vi "CSM MDI.vi"(7 "Name (\"\" to Use UUID)":string="Event CSM") -> ()   [LabVIEW 2020, in "MDI ViewManager.lvlib"]
uses:
  MDI ViewManager.lvlib
  Typedef/View.ctl
  <vilib>/Utility/miscctls.llb/LVPointTypeDef.ctl
  <vilib>/Utility/miscctls.llb/LVPoint32TypeDef.ctl
  Typedef/Layout.ctl
  <vilib>/Utility/miscctls.llb/LVBoundsTypeDef.ctl
  <vilib>/Utility/miscctls.llb/LVPositionTypeDef.ctl
  Typedef/Update View.ctl
  e08e3f9e-33cf-4499-bbf1-3a0f395d34a1.vi
  81b46446-0aca-48f9-86dc-ebdbbb8ef4b6.vi
  7ba8cf38-d999-4af7-9cb2-e6092c4454ab.vi
  5110686f-90b8-48a6-8112-abce107b1655.vi
  <userlib>/_NEVSTOP/Communicable State Machine(CSM)/AdvanceAPI/CSM - Revert Arguments-Safe String.vi
  <userlib>/_NEVSTOP/Communicable State Machine(CSM)/_Shared/Trim Single-line Text.vi
  <userlib>/_NEVSTOP/Communicable State Machine(CSM)/AdvanceAPI/CSM - Make String Arguments Safe.vi
  <userlib>/_NEVSTOP/Communicable State Machine(CSM)/AdvanceAPI/CSM - Break Down Multiple States String.vi
  <userlib>/_NEVSTOP/Communicable State Machine(CSM)/AdvanceAPI/CSM - Compact Multiple States.vi
  e08e3f9e-33cf-4499-bbf1-3a0f395d34a1.vi/b09b9099-6be0-413b-8afc-4908471460c3.vi
  <userlib>/_NEVSTOP/Communicable State Machine(CSM)/addons/INI-Static-Variable-Support/_Support/FlagInstance-CSMINIVariable.vi
  81b46446-0aca-48f9-86dc-ebdbbb8ef4b6.vi/99de0c97-112a-4c86-9094-c187659127e1.vi
  <userlib>/_NEVSTOP/Communicable State Machine(CSM)/AdvanceAPI/CSM - Keywords.vi
  <userlib>/_NEVSTOP/Communicable State Machine(CSM)/_Support/ChangeFlag/ChangeFlag-Read.vi
  <vilib>/Utility/cursorutil.llb/Set Cursor (Icon Pict).vi
  <userlib>/_NEVSTOP/Communicable State Machine(CSM)/_Support/ChangeFlag/ChangeFlagDB.vi
  <vilib>/Utility/Data Type/Get Type Information.vi
  <userlib>/_NEVSTOP/Communicable State Machine(CSM)/addons/API-String-Arugments-Support/_Support/Data To SingleElementsArray_csm.vi
  <userlib>/_NEVSTOP/Communicable State Machine(CSM)/addons/INI-Static-Variable-Support/_Support/Parse Used Session and Name.vi
  <userlib>/_NEVSTOP/Communicable State Machine(CSM)/addons/API-String-Arugments-Support/_Support/Data To API String Arguments.vi
  <userlib>/_NEVSTOP/Communicable State Machine(CSM)/addons/INI-Static-Variable-Support/_Support/INI-FGV(lvlibp).vi
  <userlib>/_NEVSTOP/Communicable State Machine(CSM)/addons/INI-Static-Variable-Support/_Support/Populate String with INI Variable.vi
  <userlib>/_NEVSTOP/Communicable State Machine(CSM)/addons/API-String-Arugments-Support/_Support/Convert API String Arguments to Data(variant).vi
  <userlib>/_NEVSTOP/Communicable State Machine(CSM)/addons/API-String-Arugments-Support/_Support/SingleElementsArray To Data_csm.vi
  <userlib>/_NEVSTOP/Communicable State Machine(CSM)/Communicable State Machine.lvlib
  <userlib>/_NEVSTOP/Communicable State Machine(CSM)/addons/INI-Static-Variable-Support/INI-Static-Variable-Support.lvlib
panel:
  in  "Tab Control 40":T1 caption="View0"
  in  "Tab Control 39":T1 caption="View1"
  in  "Tab Control 38":T1 caption="View2"
  in  "Tab Control 37":T1 caption="View3"
  in  "Tab Control 36":T1 caption="View4"
  in  "Tab Control 35":T1 caption="View5"
  in  "Tab Control 34":T1 caption="View6"
  in  "Tab Control 33":T1 caption="View7"
  in  "Tab Control 32":T1 caption="View8"
  in  "Tab Control 31":T1 caption="View9"
  in  "Tab Control 30":T1 caption="View10"
  in  "Tab Control 29":T1 caption="View11"
  in  "Tab Control 28":T1 caption="View12"
  in  "Tab Control 27":T1 caption="View13"
  in  "Tab Control 26":T1 caption="View14"
  in  "Tab Control 25":T1 caption="View15"
  in  "Tab Control 24":T1 caption="View16"
  in  "Tab Control 23":T1 caption="View17"
  in  "Tab Control 22":T1 caption="View18"
  in  "Tab Control 21":T1 caption="View19"
  in  "Tab Control 20":T1 caption="View20"
  in  "Tab Control 19":T1 caption="View21"
  in  "Tab Control 18":T1 caption="View22"
  in  "Tab Control 17":T1 caption="View23"
  in  "Tab Control 16":T1 caption="View24"
  in  "Tab Control 15":T1 caption="View25"
  in  "Tab Control 14":T1 caption="View26"
  in  "Tab Control 13":T1 caption="View27"
  in  "Tab Control 12":T1 caption="View28"
  in  "Tab Control 11":T1 caption="View29"
  in  "Tab Control 10":T1 caption="View30"
  in  "Tab Control 9":T1 caption="View31"
  in  "Tab Control 8":T1 caption="View32"
  in  "Tab Control 7":T1 caption="View33"
  in  "Tab Control 6":T1 caption="View34"
  in  "Tab Control 5":T1 caption="View35"
  in  "Tab Control 4":T1 caption="View36"
  in  "Tab Control 3":T1 caption="View37"
  in  "Tab Control 2":T1 caption="View38"
  in  "Tab Control":T1 caption="View39"
  out "State History":string
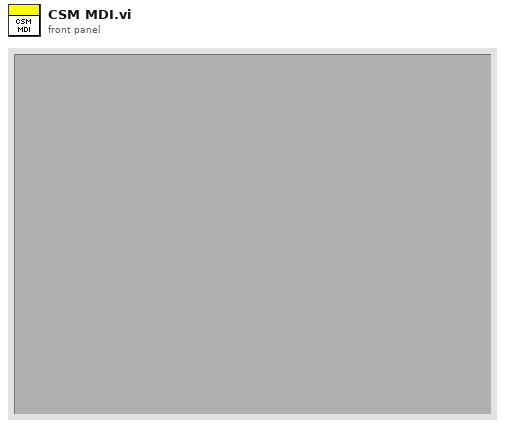
[diagram p1: front panel]
types:
  T1 = typedef "MDI ViewManager.lvlib/View.ctl" = enum32{"Page 1", "Page 2"}
  T2 = typedef "LVPointTypeDef.ctl" = cluster{"Horizontal":i16, "Vertical":i16}
  T3 = typedef "LVPoint32TypeDef.ctl" = cluster{"Horizontal":i32, "Vertical":i32}
  T4 = typedef "MDI ViewManager.lvlib/Layout.ctl" = cluster{"Origin":T2, "Layout":cluster{"Pane Dimension":T5, "Position":T6, "Label":string, "Visible":bool, "InsertedViewName":string}[]}
  T5 = typedef "LVBoundsTypeDef.ctl" = cluster{"Width":u32, "Height":u32}
  T6 = typedef "LVPositionTypeDef.ctl" = cluster{"Left":i32, "Top":i32}
  T7 = typedef "MDI ViewManager.lvlib/Update View.ctl" = cluster{"Name":string, "VIPath":path, "Height(Default)":u32, "Widht(Default)":u32, "VIRef":refnum<vi>}
  T8 = cluster{"Ref":cluster{"TabCtls":refnum<vi>[], "CurrMoveCtl":refnum<vi>, "Pane":refnum<vi>, "SubPanel":refnum<vi>, "Owning VI":refnum<vi>}, "Val":cluster{"TabCtlMove?":bool, "MouseOffset":T3, "LayoutMap":map{string, T4}, "ViewMap":map{string, T7}}}
  T9 = cluster{"Current VI Reference":refnum<vi>, "Close Panel on Exit?":bool}
  T10 = cluster{"Core":cluster{"Current VI Reference":refnum<vi>, "Close Panel on Exit?":bool}, "1":cluster{"Ref":cluster{"TabCtls":refnum<vi>[], "CurrMoveCtl":refnum<vi>, "Pane":refnum<vi>, "SubPanel":refnum<vi>, "Owning VI":refnum<vi>}, "Val":cluster{"TabCtlMove?":bool, "MouseOffset":T3, "LayoutMap":map{string, T4}, "ViewMap":map{string, T7}}}}
  T11 = enum32{"Invalid", "Standard", "Closed", "Hidden", "Minimized", "Maximized"}
  T12 = enum32{"invalid app kind", "Development System", "Run Time System", "Student Edition", "Embedded LabVIEW", "Evaluation", "Custom"}
  T13 = cluster{"TabCtl":refnum<vi>[], "Pane":refnum<vi>, "Variant":variant, "map in":map{string, T4}}
  T14 = cluster{"Pane":refnum<vi>, "TabCtls":refnum<vi>[], "map in":map{string, T4}, "Views":map{string, T7}}
  T15 = typedef "Communicable State Machine.lvlib/_CSM_Response Source Message.ctl" = cluster{"‘State":string, "’Arguments":string, "’Error":errorcluster}
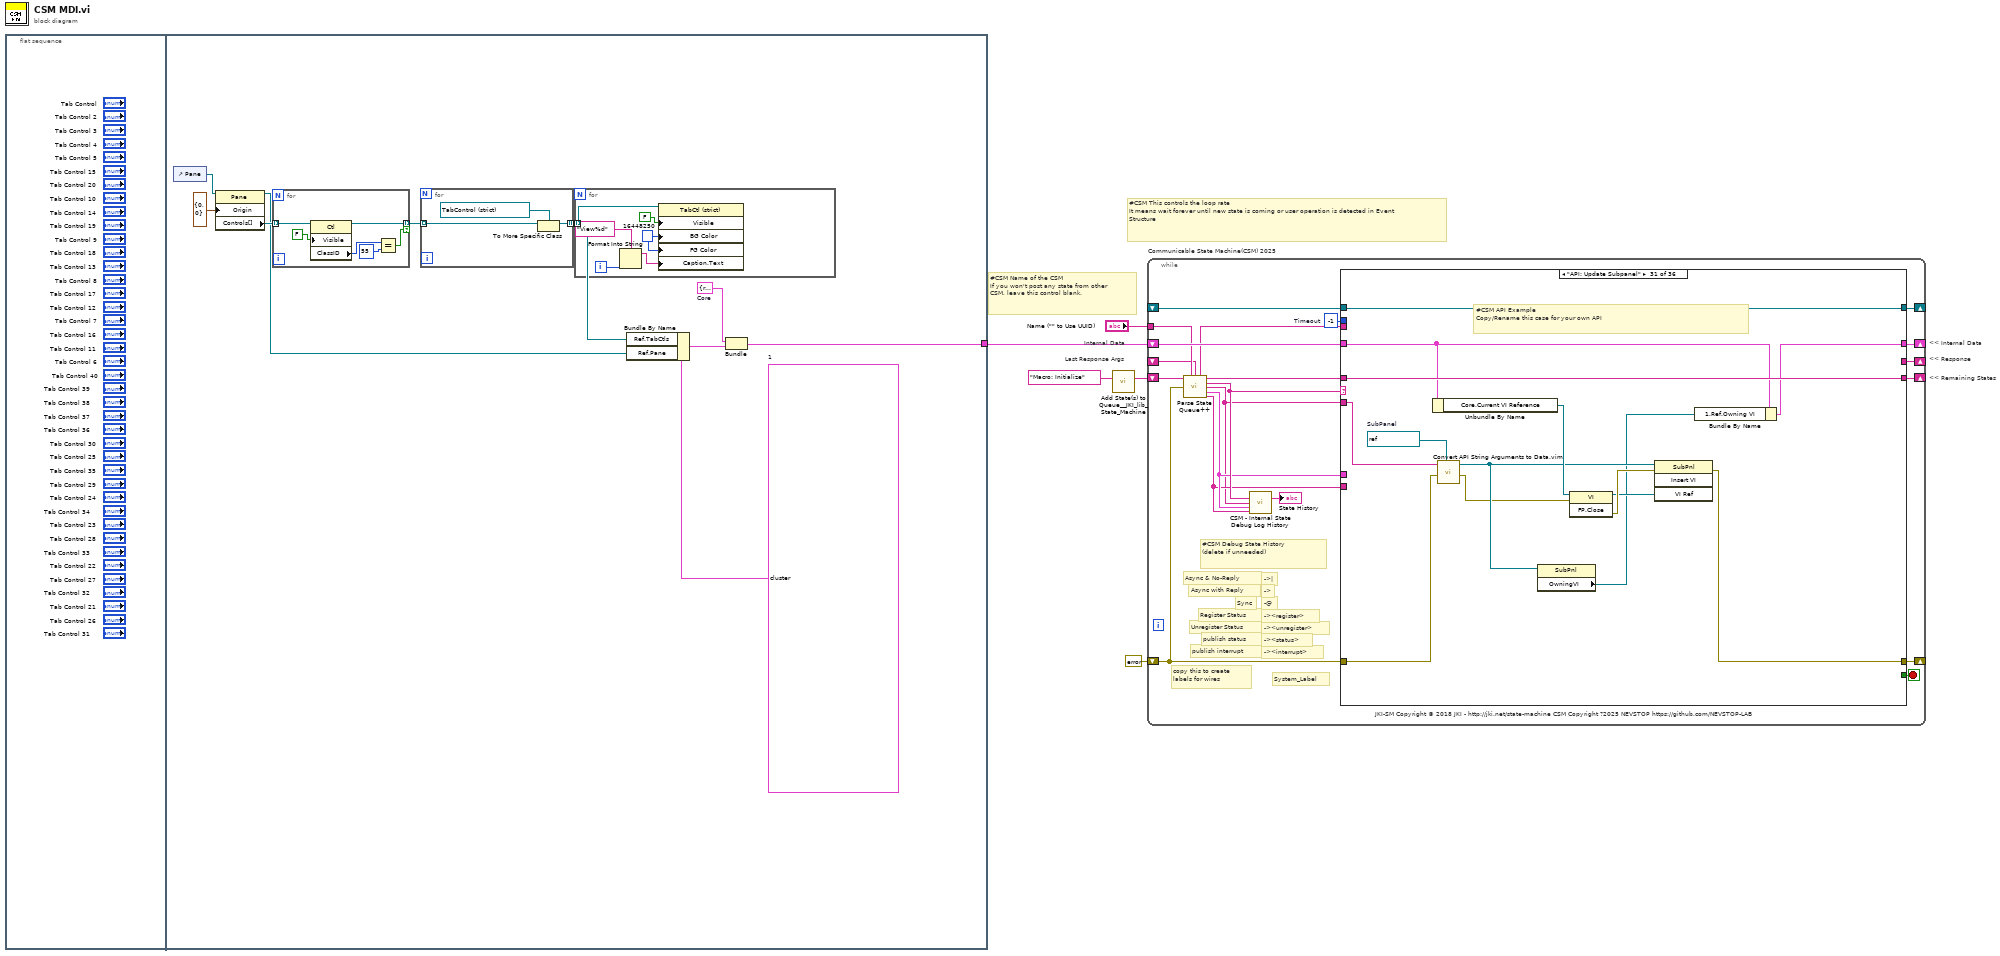
[diagram p0: block diagram]
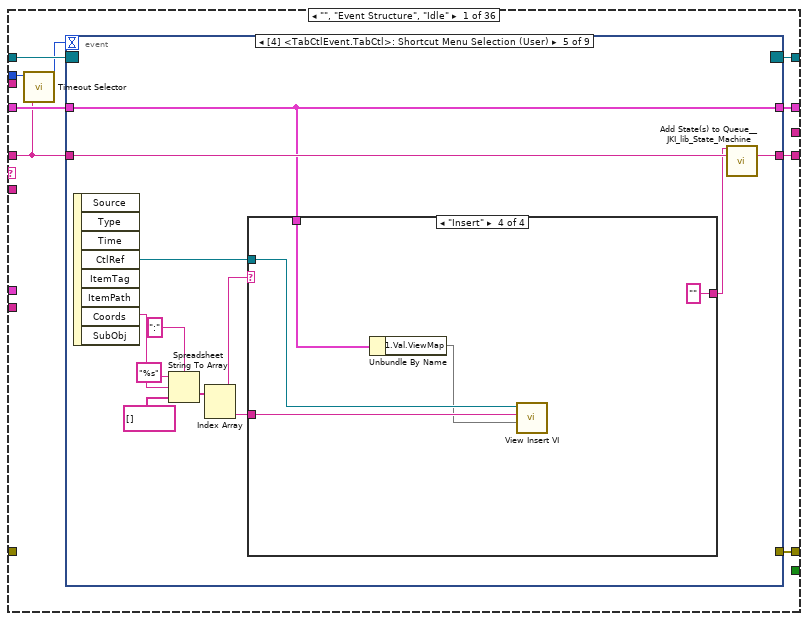
[diagram p2: hidden frame]
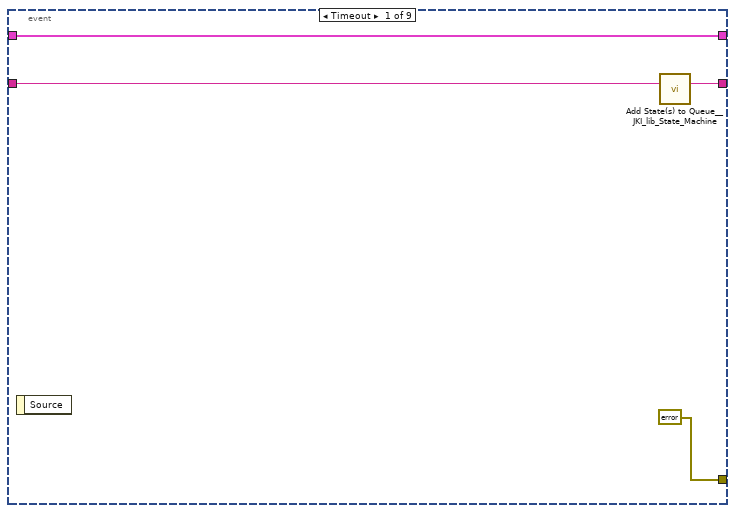
[diagram p3: hidden frame]
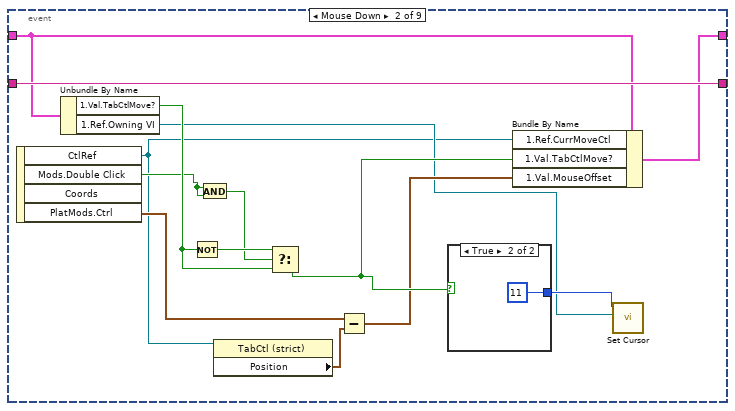
[diagram p4: hidden frame]
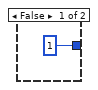
[diagram p5: hidden frame]
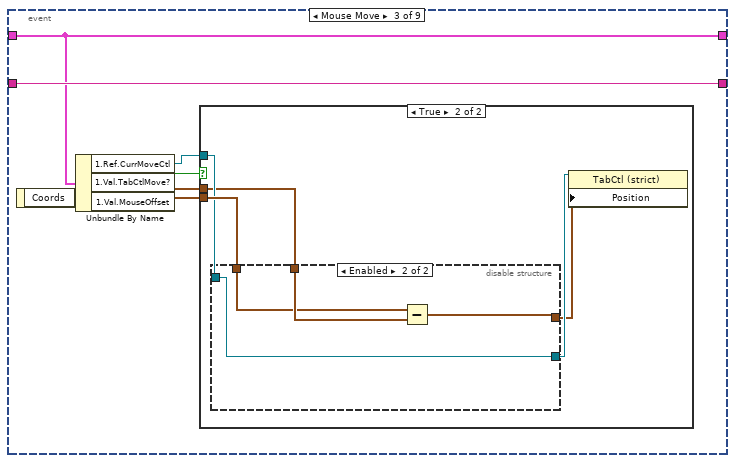
[diagram p6: hidden frame]
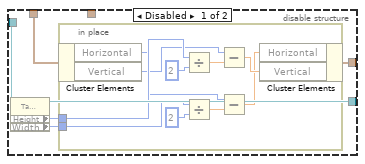
[diagram p8: hidden frame]
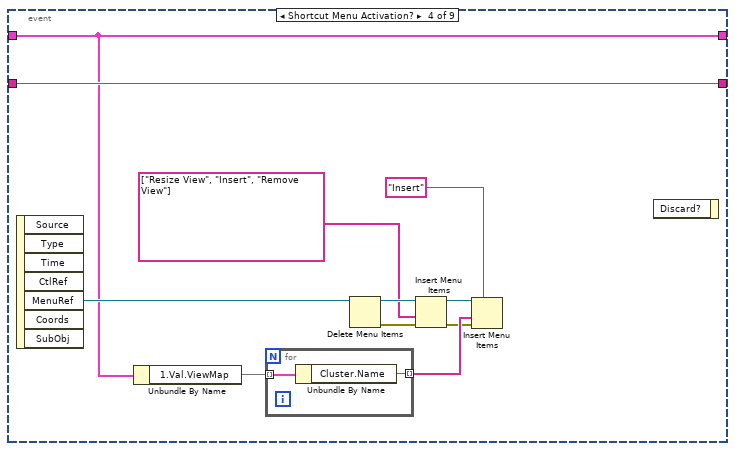
[diagram p9: hidden frame]
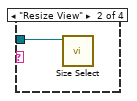
[diagram p11: hidden frame]
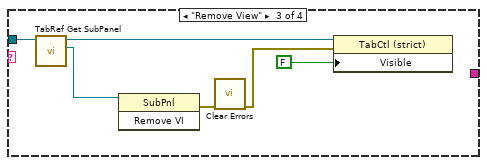
[diagram p12: hidden frame]
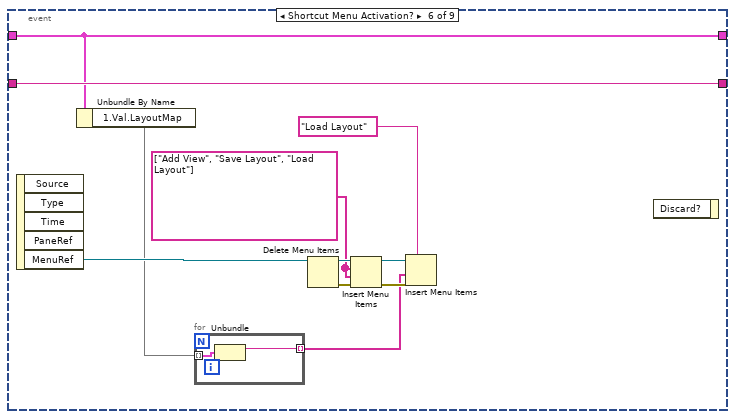
[diagram p13: hidden frame]
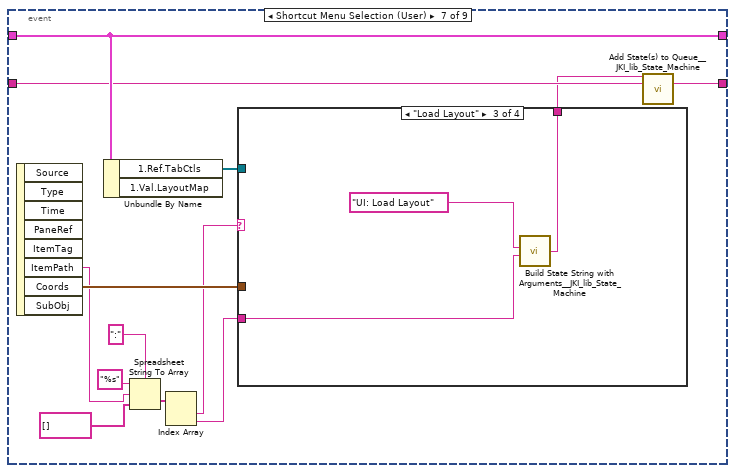
[diagram p14: hidden frame]
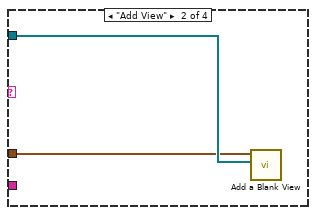
[diagram p16: hidden frame]
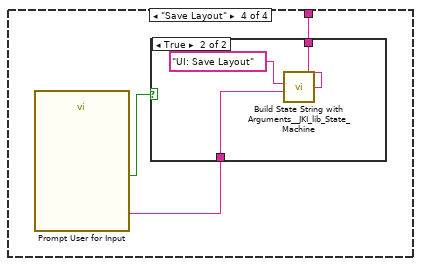
[diagram p17: hidden frame]
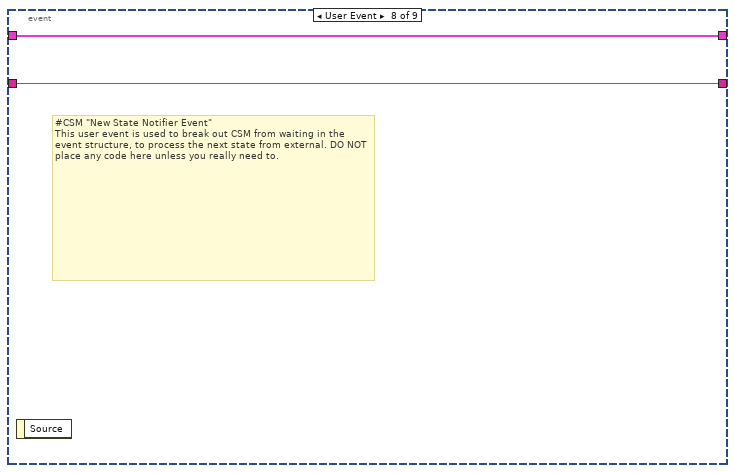
[diagram p19: hidden frame]
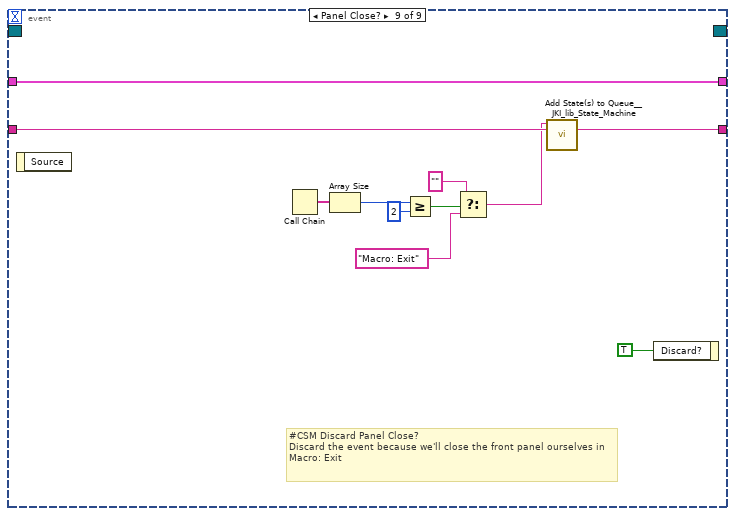
[diagram p20: hidden frame]
diagram:
  # "Last Response Args"
  # "Internal Data"
  # "<< Internal Data"
  # "<< Response"
  # "<< Remaining States"
  # "#CSM Name of the CSM\nIf you won't post any state from other CSM, leave this control blank."
  # "#CSM This controls the loop rate\nIt means wait forever until new state is coming or user operation is detected in Event Structure"
  n1 = flat-sequence {
    tunnel: [w15] -> w1
    frame #0 {
    }
    frame #1 {
      w13 = T8 {"Ref"={"TabCtls"=[], "CurrMoveCtl"=refnum, "Pane"=refnum, "SubPanel"=refnum, "Owning VI"=refnum}, "Val"={"TabCtlMove?"=FALSE, "MouseOffset"={"Horizontal"=0, "Vertical"=0}, "LayoutMap"={}, "ViewMap"={}}}  # 1
      w12 = T9 {"Current VI Reference"=refnum, "Close Panel on Exit?"=FALSE}  # Core
      n2 = control-ref of="Pane"() -> (w9:refnum<vi>)
      n3 = property class="Pane"(reference=w9, "Origin"=T2 {"Horizontal"=0, "Vertical"=0}) -> (reference out=w6:refnum<vi>, "Controls[]"=w10:refnum<vi>[])  [unwired: 1 in, 1 out]
      n4 = for {
        tunnel: w10 -> [w24] mode=indexing
        tunnel: [w19] -> w8 mode=indexing if=w20
        n5 = property class="Ctl"(reference=w24, "Visible"=FALSE) -> (reference out=w19:refnum<vi>, "ClassID"=w22:u32)  [unwired: 1 in, 1 out]
        n6 = Equal?(x=w22, y=u32 55) -> (x = y?=w20:bool)
      }
      n7 = for {
        tunnel: w8 -> [w18] mode=indexing
        tunnel: [w17] -> w7 mode=indexing
        n8 = To More Specific Class(target class=refnum<vi> refnum ("Tab Control"), reference=w18) -> (specific class reference=w17:refnum<vi>)  [unwired: 1 in, 1 out]
      }
      n9 = for {
        tunnel: w7 -> [w29] mode=indexing
        i -> [w27]
        w28 = u32 16448250 ("Colors:BG Color")
        n10 = Format Into String(format string="View%d", w27) -> (resulting string=w26:string)  [unwired: 2 in, 1 out]
        n11 = property class="TabCtl (strict)"(reference=w29, "Visible"=FALSE, "BG Color"=w28, "FG Color"=w28, "Caption.Text"=w26) -> ()  [unwired: 1 in, 2 out]
      }
      n12 = Bundle By Name(cluster=w13, "Ref.TabCtls"=w7, "Ref.Pane"=w6) -> (w14:T8)
      n13 = Bundle("Core"=w12, "1"=w14) -> (w15:T10)  [unwired: 1 in]
    }
  }
  n14 = call <vilib>:"Add State(s) to Queue__JKI_lib_State_Machine.vi"("State(s) in (\"\")"="Macro: Initialize" ("Init State(\"Macro: Initialize\")")) -> ("States Out"=w2:string)  [unwired: 14 in]
  n15 = while "Communicable State Machine(CSM) 2025" {
    shift-right: [w45] -> _
    shift-left: w1 -> [w44]
    shift-right: [w48] -> _
    shift-left: errorcluster {"status"=FALSE, "code"=0, "source"=""} ("error out") -> [w42]
    shift-right: [w47] -> _
    shift-left: w2 -> [w49]
    tunnel: "Name (\"\" to Use UUID)" -> [w38]
    shift-right: [w41] -> _
    shift-left: _ -> [w33]
    shift-right: [w40] -> _
    shift-left: _ -> [w39]
    stop <- w46 stop-if-true
    w43 = -1  # Timeout
    # "#CSM Debug State History\n(delete if unneeded)"
    # "-><interrupt>"
    # "-><status>"
    # "-><unregister>"
    # "-><register>"
    # "-@"
    # "->"
    # "->|"
    # "publish interrupt"
    # "publish status"
    # "Unregister Status"
    # "Register Status"
    # "Sync"
    # "Async with Reply"
    # "Async & No-Reply"
    # "copy this to create labels for wires"
    # "System_Label"
    # "JKI-SM Copyright © 2018 JKI - http://jki.net/state-machine CSM Copyright ?2025 NEVSTOP https://github.com/NEVSTOP-LAB"
    n16 = call <userlib>:"Parse State Queue++.vi"("State Queue"=w49, "Name (\"\" to Use UUID)"=w38, "Response Arguments"=w33, "Previous Error"=w42) -> ("Name Used"=w34:string, "Remaining States"=w50:string, "Current State"=w37:string, "Arguments"=w32:string, "Additional Information"=w36:T15, "Source CSM"=w35:string)  [unwired: 6 in]
    n17 = call <userlib>:"CSM - Internal State Debug Log History.vi"("State"=w37, "Arguments (\"\")"=w32, ">> Response Source Message >>"=w36, "Source (\"\")"=w35) -> ("Debug Log"=→"State History":string)  [unwired: 11 in]
    n18 = case shown="\"API: Update Subpanel\"" w37 {
      selector: w37 -> [_ _ _ w208 _ _ _ _ _ _ _ _ _ _ _ _ _ _ _ _ _ _ _ _ _ _ _ _ _ _ _ _ _ _ _ _]
      tunnel: w50 -> [w52 w200 w205 w214 w220 w226 w252 w260 w267 w277 w286 w299 w304 w308 w316 w330 w337 w347 w351 w355 w359 w372 w384 w390 w401 w465 w470 w481 w484 w494 w508 w511 w519 w528 w532 w536]
      tunnel: w32 -> [_ _ _ _ _ w224 w248 w255 w263 w271 _ _ _ _ _ _ _ _ _ _ _ w368 w378 w386 w396 _ _ _ _ w485 w496 w512 w520 _ _ _]
      tunnel: w44 -> [w58 w199 w202 w212 w219 w232 w253 w258 w265 w275 w285 w293 w302 w306 w313 w326 w335 w339 w350 w353 w356 w367 w382 w388 w398 w463 w468 w479 w483 w492 w504 w516 w524 w526 w530 w534]
      tunnel: [w57 _ w203 w206 w221 errorcluster {"status"=FALSE, "code"=0, "source"=""} ("error out") w245 w254 w261 w274 _ _ _ _ _ w327 _ w342 w349 _ _ w369 w376 w387 w399 _ _ _ _ _ w497 w513 w521 _ _ _] -> w48
      tunnel: w42 -> [_ _ w203 w207 w221 w230 w246 w256 w262 _ _ _ _ _ _ w324 _ _ _ _ _ w370 w377 _ _ _ _ _ _ _ w499 w513 w521 _ _ _]
      tunnel: [w59 w200 w204 w213 w220 w228 w251 w259 w266 w278 w286 w298 w303 w307 w315 w329 w336 w347 w351 w354 w358 w372 w384 w389 w400 w464 w469 w480 w484 w494 w508 w510 w518 w527 w531 w535] -> w47
      tunnel: [_ _ _ _ _ _ TRUE _ _ _ _ _ TRUE _ _ _ _ _ _ _ _ _ _ _ _ _ _ _ _ _ _ _ _ _ _ _] -> w46
      tunnel: [w56 w199 w202 w212 w219 w232 w253 w258 w265 w276 w285 w297 w302 w306 w310 w326 w335 w339 w350 w353 w356 w361 w382 w388 w398 w463 w468 w479 w483 w490 w502 w516 w524 w526 w530 w534] -> w45
      tunnel: w43 -> [w54 _ _ _ _ _ _ _ _ _ _ _ _ _ _ _ _ _ _ _ _ _ _ _ _ _ _ _ _ _ _ _ _ _ _ _]
      tunnel: w35 -> [_ _ _ _ _ w223 _ _ _ w272 _ _ _ _ _ _ _ _ _ _ _ _ _ _ _ _ _ _ _ _ _ _ _ _ _ _]
      tunnel: w36 -> [_ _ _ _ _ w222 _ _ _ w273 _ _ _ _ _ _ _ _ _ _ _ _ _ _ _ _ _ _ _ _ _ _ _ _ _ _]
      tunnel: [_ _ _ "" w215 _ _ _ _ _ _ _ _ _ _ _ _ _ _ _ _ _ _ _ _ _ _ _ _ _ _ _ _ _ _ _] -> w41
      tunnel: [w51 w198 w201 w210 w218 w231 w249 w257 w264 w279 w284 w287 w300 w305 w314 w325 w334 w346 w348 w352 w357 w371 w383 w385 w395 w462 w466 w472 w482 w493 w507 w515 w523 w525 w529 w533] -> w40
      tunnel: w39 -> [w55 w198 w201 w210 w218 w231 w249 w257 w264 w279 w284 w287 w300 w305 w314 w325 w334 _ w348 w352 w357 w371 w383 w385 w395 w462 w466 w472 w482 w493 w507 w515 w523 w525 w529 w533]
      tunnel: w34 -> [_ _ _ w209 _ _ w247 _ _ _ _ _ _ _ w311 w320 _ w345 _ _ _ _ _ _ _ _ _ _ _ _ _ _ _ _ _ _]
      frame "", "Event Structure", "Idle" {
        n19 = call <userlib>:"Timeout Selector.vi"("Remaining States"=w52, "Timeout Expected"=w54) -> ("Timeout"=w53:i32)  [unwired: 5 in]
        n20 = event shown="[4] <TabCtlEvent.TabCtl>: Shortcut Menu Selection (User)" {
          selector: w55 -> [_ _ _ _ _ _ _ _ _]
          dyn-events: [_ _ _ _ _ _ _ _ _] -> w51
          timeout: w53 -> [_ _ _ _ _ _ _ _ _]
          tunnel: w52 -> [w63 w77 w85 w121 w134 w158 w171 w185 w197]
          tunnel: [w62 w77 w85 w121 w133 w158 w170 w185 w196] -> w59
          tunnel: w58 -> [w61 w74 w83 w115 w124 w153 w173 w186 w195]
          tunnel: [errorcluster {"status"=FALSE, "code"=0, "source"=""} ("error out") _ _ _ _ _ _ _ _] -> w57
          tunnel: [w61 w72 w83 w115 w124 w153 w173 w186 w195] -> w56
          event Timeout {
            n21 = event-data() -> ()  [unwired: 1 in, 1 out]
            n22 = call <vilib>:"Add State(s) to Queue__JKI_lib_State_Machine.vi"("State(s) in (\"\")"=w63) -> ("States Out"=w62:string)  [unwired: 14 in]
          }
          event Mouse Down {
            n23 = event-data() -> ("CtlRef"=w64:refnum<vi>, "Mods.Double Click"=w65:bool, "Coords"=w69:T3)  [unwired: 1 in, 1 out]
            n24 = Unbundle By Name(w74) -> ("1.Val.TabCtlMove?"=w73:bool, "1.Ref.Owning VI"=w67:refnum<vi>)
            n25 = Not(x=w73) -> (.not. x?=w76:bool)
            n26 = And(x=w65, y=w65) -> (x .and. y?=w66:bool)
            n27 = property class="TabCtl (strict)"(reference=w64) -> ("Position"=w70:T6)  [unwired: 1 in, 2 out]
            n28 = Select(t=w76, s=w66, f=w73) -> (s? t:f=w71:bool)
            n29 = Subtract(x=w69, y=w70) -> (x-y=w68:T3)
            n30 = case shown="True" w71 {
              tunnel: [u16 1 ("icon") u16 11 ("icon")] -> w75
              frame False {
              }
              frame True {
              }
            }
            n31 = Bundle By Name(cluster=w74, "1.Ref.CurrMoveCtl"=w64, "1.Val.TabCtlMove?"=w71, "1.Val.MouseOffset"=w68) -> (w72:T10)
            n32 = call-poly <vilib>:"Set Cursor.vi"("VI reference (current VI)"=w67, "icon"=w75) -> ()  [unwired: 8 in, 2 out]
          }
          event Mouse Move {
            n33 = event-data() -> ("Coords"=w84:T3)  [unwired: 1 in]
            n34 = Unbundle By Name(w83) -> ("1.Ref.CurrMoveCtl"=w81:refnum<vi>, "1.Val.TabCtlMove?"=w82:bool, "1.Val.MouseOffset"=w80:T3)
            n35 = case shown="True" w82 {
              tunnel: w84 -> [_ w90]
              tunnel: w81 -> [_ w89]
              tunnel: w80 -> [_ w86]
              frame False {
              }
              frame True {
                n36 = disable-structure shown="Enabled" {
                  disable-tunnel: w90 -> [w94 w108]
                  disable-tunnel: w89 -> [w93 w110]
                  disable-tunnel: [w92 w110] -> w88
                  disable-tunnel: [w91 w107] -> w87
                  disable-tunnel: w86 -> [_ w109]
                  frame Disabled {
                    n37 = property class="TabCtl (strict)"(reference=w93) -> (reference out=w92:refnum<vi>, "Height"=w96:u32, "Width"=w95:u32)  [unwired: 1 in, 1 out]
                    n38 = in-place {
                      in-place-border: w96 -> [w106]
                      in-place-border: w95 -> [w100]
                      n39 = in-place-cluster #1(w94) -> ("Horizontal"=w98:i32, "Vertical"=w97:i32)
                      n40 = Divide(x=w106, y=u32 2) -> (x/y=w104:dbl)
                      n41 = Divide(x=w100, y=u32 2) -> (x/y=w101:dbl)
                      n42 = Subtract(x=w97, y=w104) -> (x-y=w103:dbl)
                      n43 = Subtract(x=w98, y=w101) -> (x-y=w99:dbl)
                      n44 = in-place-cluster #1("Horizontal"=w99, "Vertical"=w103) -> (w91:T3)
                    }
                  }
                  frame Enabled {
                    n45 = Subtract(x=w108, y=w109) -> (x-y=w107:T3)
                  }
                }
                n46 = property class="TabCtl (strict)"(reference=w88, "Position"=w87) -> ()  [unwired: 1 in, 2 out]
              }
            }
          }
          event Shortcut Menu Activation? {
            n47 = event-data() -> ("MenuRef"=w117:refnum<k9>)  [unwired: 1 in, 6 out]
            n48 = Unbundle By Name(w115) -> ("1.Val.ViewMap"=w114:map{string, T7})
            n49 = for {
              tunnel: w114 -> [w123] mode=indexing
              tunnel: [w122] -> w113 mode=indexing
              n50 = Unbundle By Name(w123) -> ("Cluster.Name"=w122:string)
            }
            n51 = Delete Menu Items(9:w117) -> (0:w120:errorcluster, 3:w119:refnum<k9>)  [unwired: 3 in]
            n52 = Insert Menu Items(6:w120, 7:string[] ["Resize View", "Insert", "Remove View"] ("item names"), 9:w119) -> (0:w111:errorcluster, 3:w112:refnum<k9>)  [unwired: 3 in, 1 out]
            n53 = Insert Menu Items(5:"Insert", 6:w111, 7:w113, 9:w112) -> ()  [unwired: 2 in, 3 out]
            n54 = event-data() -> ()  [unwired: 2 in, 1 out]
          }
          event Shortcut Menu Selection (User) {
            n55 = event-data() -> ("CtlRef"=w135:refnum<vi>, "ItemPath"=w130:string)  [unwired: 1 in, 6 out]
            n56 = Spreadsheet String To Array(delimiter (Tab)=":", format string="%s", spreadsheet string=w130, array type (2D Dbl)=string[] [] ("delimiter (Tab)")) -> (array=w127:string[])
            n57 = Index Array(array=w127) -> (element #1=w126:string, element #2=w125:string)  [unwired: 2 in]
            n58 = case shown="\"Insert\"" w126 {
              tunnel: w135 -> [_ w136 w142 w145]
              tunnel: [_ _ _ "" ("State(s) in Front (\"\")")] -> w132
              tunnel: w125 -> [_ _ _ w146]
              tunnel: w124 -> [_ _ _ w147]
              frame "False", Default {
              }
              frame "Resize View" {
                n59 = call "Size Select.vi"("CtlRef"=w136) -> ()  [unwired: 11 in]
              }
              frame "Remove View" {
                n60 = call "TabRef Get SubPanel.vi"("TabControl in"=w142) -> ("Sub Panel"=w138:refnum<vi>, "TabControl out"=w141:refnum<vi>)  [unwired: 8 in, 1 out]
                n61 = invoke class="SubPnl" method="Remove VI"(reference=w138) -> (error out=w139:errorcluster)  [unwired: 2 in, 2 out]
                n62 = call <vilib>:"Clear Errors.vi"("error in (no error)"=w139) -> ("error out"=w137:errorcluster)  [unwired: 5 in, 1 out]
                n63 = property class="TabCtl (strict)"(reference=w141, error in=w137, "Visible"=FALSE) -> ()  [unwired: 2 out]
              }
              frame "Insert" {
                n64 = Unbundle By Name(w147) -> ("1.Val.ViewMap"=w143:map{string, T7})
                n65 = call "View Insert VI.vi"("ViewMap"=w143, "Name"=w146, "TabControl in"=w145) -> ()  [unwired: 7 in, 2 out]
              }
            }
            n66 = call <vilib>:"Add State(s) to Queue__JKI_lib_State_Machine.vi"("State(s) in Front (\"\")"=w132, "State(s) in (\"\")"=w134) -> ("States Out"=w133:string)  [unwired: 13 in]
          }
          event Shortcut Menu Activation? {
            w155 = string[] ["Add View", "Save Layout", "Load Layout"] ("item names")
            n67 = event-data() -> ("MenuRef"=w154:refnum<k9>)  [unwired: 1 in, 4 out]
            n68 = Unbundle By Name(w153) -> ("1.Val.LayoutMap"=w152:map{string, T4})
            n69 = for {
              tunnel: w152 -> [w160] mode=indexing
              tunnel: [w159] -> w149 mode=indexing
              n70 = Unbundle(w160) -> (w159:string)  [unwired: 1 out]
            }
            n71 = Delete Menu Items(9:w154) -> (0:w157:errorcluster, 3:w156:refnum<k9>)  [unwired: 3 in]
            n72 = Insert Menu Items(6:w157, 7:w155, 8:w155, 9:w156) -> (0:w151:errorcluster, 3:w150:refnum<k9>)  [unwired: 2 in, 1 out]
            n73 = Insert Menu Items(5:"Load Layout", 6:w151, 7:w149, 9:w150) -> ()  [unwired: 2 in, 3 out]
            n74 = event-data() -> ()  [unwired: 2 in, 1 out]
          }
          event Shortcut Menu Selection (User) {
            n75 = event-data() -> ("ItemPath"=w164:string, "Coords"=w168:T3)  [unwired: 1 in, 6 out]
            n76 = Unbundle By Name(w173) -> ("1.Ref.TabCtls"=w172:refnum<vi>[])  [unwired: 1 out]
            n77 = Spreadsheet String To Array(delimiter (Tab)=":", format string="%s", spreadsheet string=w164, array type (2D Dbl)=string[] [] ("delimiter (Tab)")) -> (array=w165:string[])
            n78 = Index Array(array=w165) -> (element #1=w162:string, element #2=w161:string)  [unwired: 2 in]
            n79 = case shown="\"Load Layout\"" w162 {
              tunnel: w172 -> [_ w175 _ _]
              tunnel: w168 -> [_ w174 _ _]
              tunnel: [_ _ w176 w181] -> w169
              tunnel: w161 -> [_ _ w177 _]
              frame "False", Default {
              }
              frame "Add View" {
                n80 = call "Add a Blank View.vi"("TabCtls"=w175, "Coords"=w174) -> ()  [unwired: 9 in, 1 out]
              }
              frame "Load Layout" {
                n81 = call <vilib>:"Build State String with Arguments__JKI_lib_State_Machine.vi"("Arguments (\"\")"=w177, "State"="UI: Load Layout" ("State(s) in Front (\"\")")) -> ("State with Arguments"=w176:string)  [unwired: 4 in]
              }
              frame "Save Layout" {
                n82 = call "Prompt User for Input"() -> ("name"=w180:string, "OK"=w179:bool)  [unwired: 17 in, 1 out]
                n83 = case shown="True" w179 {
                  tunnel: [_ w183] -> w181
                  tunnel: w180 -> [_ w182]
                  frame False {
                  }
                  frame True {
                    n84 = call <vilib>:"Build State String with Arguments__JKI_lib_State_Machine.vi"("Arguments (\"\")"=w182, "State"="UI: Save Layout" ("State(s) in Front (\"\")")) -> ("State with Arguments"=w183:string)  [unwired: 4 in]
                  }
                }
              }
            }
            n85 = call <vilib>:"Add State(s) to Queue__JKI_lib_State_Machine.vi"("State(s) in Front (\"\")"=w169, "State(s) in (\"\")"=w171) -> ("States Out"=w170:string)  [unwired: 13 in]
          }
          event User Event {
            # "#CSM \"New State Notifier Event\"\nThis user event is used to break out CSM from waiting in the event structure, to process the next state from external. DO NOT place any code here unless you really need to."
            n86 = event-data() -> ()  [unwired: 1 in, 1 out]
          }
          event Panel Close? {
            # "#CSM Discard Panel Close?\nDiscard the event because we'll close the front panel ourselves in Macro: Exit"
            n87 = event-data() -> ()  [unwired: 1 in, 1 out]
            n88 = Call Chain() -> (call chain=w188:string[])
            n89 = Array Size(array=w188) -> (size(s)=w193:i32)
            n90 = Greater Or Equal?(x=w193, y=2) -> (x >= y?=w191:bool)
            n91 = Select(t="", s=w191, f="Macro: Exit") -> (s? t:f=w187:string)
            n92 = call <vilib>:"Add State(s) to Queue__JKI_lib_State_Machine.vi"("State(s) in Front (\"\")"=w187, "State(s) in (\"\")"=w197) -> ("States Out"=w196:string)  [unwired: 13 in]
            n93 = event-data("Discard?"=TRUE) -> ()  [unwired: 1 in, 1 out]
          }
        }
      }
      frame "CSM Documentation" {
        # "#CSM State Syntax\n\n// Comment line, all text to the right of “//” will be ignored\n// Local Message Example\nDoSth: DoA >> Arguments\n\n// Sync Call Example\nAPI: xxxx >> Arguments -@ TargetModule\n\n// Async Call Example\nAPI: xxxx >> Arguments -> TargetModule\n\n// Async Call without Reply Example\nAPI: xxxx >> Arguments ->| TargetModule\n\n// Broadcast normal status:\nStatus >> StatusArguments  -><status>\n\n// Broadcast Interrupt status:\nInterrupt >> StatusArguments  -><interrupt>\n\n// Register Source Module's status to Handler Module\nStatus@Source Module >> Handler Module@Handler Module -><register>\n\n// Unegister Source Module's status\nStatus@Source Module >> Handler Module -><unregister>"
        # "#CSM README FIRST\n\nCommunicable State Machine(CSM) is a LabVIEW application framework that builds upon JKI State Machine(JKISM). It follows the pattern of JKISM and extends the keywords to describe message communication between modules, including concepts such as Sync-Message, Async-Message, Subscription/Unsubscription of status - essential elements for creating reusable code modules. For more information, please visit the CSM wiki: https://nevstop-lab.github.io/CSM-Wiki/\n\nFor instructions on JKI State Machine, visit: \n    http://jki.net/state-machine/\nFor information about CSM, visit: \n    https://github.com/NEVSTOP-LAB"
        # "#CSM \"Documentation\"\nCase for holding CSM Documenation"
      }
      frame "---------- Core ----------" {
        # "#CSM \"Category Seperator\"\nDo not put any code in this frame."
        n94 = call <vilib>:"Add State(s) to Queue__JKI_lib_State_Machine.vi"("State(s) in (\"\")"=w205) -> ("States Out"=w204:string)  [unwired: 14 in]
      }
      frame Default {
        # "#CSM \"Default\"\nthis is used to capture unhandled states and typos"
        n95 = call <userlib>:"CSM Unhandled State Error.vi"("error in (no error)"=w207, "Undefined State"=w208, "CSM Name"=w209) -> ("error out"=w206:errorcluster)  [unwired: 8 in]
        n96 = call <vilib>:"Add State(s) to Queue__JKI_lib_State_Machine.vi"("State(s) in (\"\")"=w214) -> ("States Out"=w213:string)  [unwired: 14 in]
      }
      frame "VI Reference" {
        n97 = Unbundle By Name(w219) -> ("Core"=w217:T9)
        n98 = Unbundle By Name(w217) -> ("Current VI Reference"=w216:refnum<vi>)
        n99 = call <userlib>:"CSM - Convert Data to HexStr.vi"("Variant"=w216) -> ("HEX String (0-9,A-F)"=w215:string)  [unwired: 8 in]
      }
      frame "Error Handler" {
        # "#CSM Disable this error dialog if you need"
        # "#CSM \"Error Handler\"\nYou can also output any states to clean-up after errors occur"
        # "Clear error"
        n100 = case shown="Error" w230 {
          selector: w230 -> [_ w239]
          tunnel: [w237 w241] -> w227
          tunnel: w226 -> [w237 w240]
          tunnel: [w236 w239] -> w225
          tunnel: w224 -> [w238 _]
          tunnel: w223 -> [_ _]
          tunnel: w222 -> [_ _]
          frame No Error {
            n101 = call <userlib>:"CSM - Convert Argument to Error.vi"("Argument"=w238) -> ("Error"=w236:errorcluster)  [unwired: 4 in]
            n102 = flat-sequence {
              frame #0 {
                # "#CSM External Error Handler Case\nUsually, it's because This CSM register others' \"Error Occurred\" status with \"Error Handler\". If other CSM have any error, the error will be passed here for central handling."
              }
            }
          }
          frame Error {
            # "#CSM Internal Error Handler Case \nIf any error Occurred, \"Error Occurred\" \nstatus update will be broadcasted to system.\nParameter is Error Cluster."
            n103 = call <userlib>:"CSM - Convert Error to Argument.vi"("Error"=w239) -> ("Argument"=w243:string)  [unwired: 4 in]
            n104 = call <vilib>:"Build State String with Arguments__JKI_lib_State_Machine.vi"("Arguments (\"\")"=w243, "State"="Error Occurred" ("Status with Arguments")) -> ("State with Arguments"=w242:string)  [unwired: 4 in]
            n105 = call <userlib>:"CSM - Broadcast Status Change.vi"("Status With Arguments"=w242, "State Queue"=w240) -> ("Remaining States"=w241:string)  [unwired: 13 in]
          }
        }
        n106 = disable-structure shown="Enabled" {
          disable-tunnel: w225 -> [w234 w235]
          frame Enabled {
            # "Unhandled Error -- Display it"
            n107 = call <vilib>:"General Error Handler.vi"("error in (no error)"=w234) -> ()  [unwired: 10 in, 5 out]
          }
          frame Disabled {
            n108 = call <vilib>:"Clear Errors.vi"("error in (no error)"=w235) -> ()  [unwired: 5 in, 2 out]
          }
        }
        n109 = call <vilib>:"Add State(s) to Queue__JKI_lib_State_Machine.vi"("State(s) in Front (\"\")"="// Post Error States", "State(s) in (\"\")"=w227) -> ("States Out"=w228:string)  [unwired: 13 in]
      }
      frame "Critical Error" {
        # "#CSM \"Critical Error\"\nWhen any un-recoverable error occurs, CSM goes into this case."
        # "#CSM Stop in Critical Error\nWhen Critical Error occurs, Stop the loop immediately. Do NOT change this unless you fully understand the impact."
        n110 = call <userlib>:"CSM Critical Error.vi"("error in (no error)"=w246, "Arugments (As Reason)"=w248, "CSM Name"=w247) -> ("error out"=w245:errorcluster)  [unwired: 8 in]
        n111 = call <vilib>:"Add State(s) to Queue__JKI_lib_State_Machine.vi"("State(s) in (\"\")"=w252) -> ("States Out"=w251:string)  [unwired: 14 in]
      }
      frame "Target Timeout Error" {
        # "#CSM \"Target Timeout Error\"\nWhen This CSM could not get the sync-call response in time, This CSM goes into this case."
        n112 = call <userlib>:"CSM Target Timeout Error.vi"("error in (no error)"=w256, "Arguments (As CSM Name)"=w255) -> ("error out"=w254:errorcluster)  [unwired: 9 in]
        n113 = call <vilib>:"Add State(s) to Queue__JKI_lib_State_Machine.vi"("State(s) in (\"\")"=w260) -> ("States Out"=w259:string)  [unwired: 14 in]
      }
      frame "Target Error" {
        # "#CSM \"Target Error\"\nWhen This CSM try to communicate with an un-existed CSM, This CSM goes into this case."
        n114 = call <userlib>:"CSM Target Error.vi"("error in (no error)"=w262, "Arguments (As CSM Name)"=w263) -> ("error out"=w261:errorcluster)  [unwired: 9 in]
        n115 = call <vilib>:"Add State(s) to Queue__JKI_lib_State_Machine.vi"("State(s) in (\"\")"=w267) -> ("States Out"=w266:string)  [unwired: 14 in]
      }
      frame "Async Response", "Response" {
        # "#CSM \"Async Response\"\nHandle Async-call Response (\"Async Response\" for ->)"
        # "#CSM \"Response\"\nHandle Sync-call Response (\"Response\" for -@)"
        n116 = Unbundle(w273) -> ("‘State"=w270:string, "’Arguments"=w269:string, "’Error"=w268:errorcluster)
        n117 = case shown="Default" w270 {
          tunnel: [w280] -> w278
          tunnel: w277 -> [w281]
          tunnel: [w283] -> w276
          tunnel: w275 -> [w283]
          tunnel: [w282] -> w274
          tunnel: w268 -> [w282]
          tunnel: w272 -> [_]
          tunnel: w271 -> [_]
          tunnel: w269 -> [_]
          frame Default {
            # "#CSM Response Comments\nAfter Message is executed, CSM goes to this state for receive the response.\n    For Async Message(->), \"Async Response\" is used. This CSM will goes to \"Async Message Posted\" immediately and receive the \"Async Response\" after the callee finishes the message.\n    For Sync Message(@),  This CSM will wait until the message is done and immediately goes to \"Response\""
            n118 = call <vilib>:"Add State(s) to Queue__JKI_lib_State_Machine.vi"("State(s) in (\"\")"=w281) -> ("States Out"=w280:string)  [unwired: 14 in]
          }
        }
      }
      frame "Async Message Posted" {
        # "#CSM \"Async Message Posted\"\nAfter Async Message is posted (-> or ->| ), CSM goes to this state for post-action.\nYou can use Argument - State to tell which Async Message is called."
      }
      frame "Initialize Core Data" {
        # "#CSM \"Initialize Core Data\"\nThis is used to determine panel behavior on exit"
        # "originally closed?"
        # "exe?"
        # "If panel starts closed or is an EXE, then close it when we exit"
        n119 = property class="VI"() -> ("FP.State"=w290:T11)  [unwired: 2 in, 2 out]
        n120 = property class="App"() -> ("App.Kind"=w296:T12)  [unwired: 2 in, 2 out]
        n121 = control-ref of="Current VI Reference"() -> (w291:refnum<vi>)
        n122 = Equal?(x=w290, y=T11."Closed" ("Front Panel Window:State")) -> (x = y?=w288:bool)
        n123 = Equal?(x=w296, y=T12."Run Time System" ("Application:Kind")) -> (x = y?=w294:bool)
        n124 = Or(x=w288, y=w294) -> (x .or. y?=w292:bool)
        n125 = Bundle By Name(cluster=w293, "Core.Current VI Reference"=w291, "Core.Close Panel on Exit?"=w292) -> (w297:T10)
        n126 = call <vilib>:"Add State(s) to Queue__JKI_lib_State_Machine.vi"("State(s) in (\"\")"=w299) -> ("States Out"=w298:string)  [unwired: 14 in]
      }
      frame "Exit" {
        # "#CSM \"Exit\"\nCase for exiting the loop. No errors that occur here will be handled."
        n127 = call <vilib>:"Add State(s) to Queue__JKI_lib_State_Machine.vi"("State(s) in (\"\")"=w304) -> ("States Out"=w303:string)  [unwired: 14 in]
      }
      frame "---------- Data ----------" {
        # "#CSM \"Category Seperator\"\nDo not put any code in this frame."
        n128 = call <vilib>:"Add State(s) to Queue__JKI_lib_State_Machine.vi"("State(s) in (\"\")"=w308) -> ("States Out"=w307:string)  [unwired: 14 in]
      }
      frame "Data: Initialize" {
        n129 = Unbundle By Name(w313) -> ("1.Val.LayoutMap"=w312:map{string, T4})
        n130 = call "CSM - Read Configuration Variable.vim"("Section Name (\"\" as Default)"=w311, "Configuration Prototype (Cluster Prefered)"=w312) -> ("Configuration"=w309:map{string, T4})  [unwired: 6 in, 1 out]
        n131 = Bundle By Name(cluster=w313, "1.Val.LayoutMap"=w309) -> (w310:T10)
        n132 = call <vilib>:"Add State(s) to Queue__JKI_lib_State_Machine.vi"("State(s) in (\"\")"=w316) -> ("States Out"=w315:string)  [unwired: 14 in]
      }
      frame "Data: Cleanup" {
        w319 = TRUE ("All Temp Variable to Default Ini(F)")
        # "#CSM \"Data: Cleanup\"\nCleanup any data and references, here.\n(this is called automatically, by the Macro: Exit)"
        n133 = Unbundle By Name(w326) -> ("Core.Current VI Reference"=w328:refnum<vi>, "1.Ref.TabCtls"=w323:refnum<vi>[], "1.Val.LayoutMap"=w321:map{string, T4})
        n134 = call "CSM - Write Configuration Variable.vim"("Section Name (\"\" as Default)"=w320, "Configuration"=w321) -> ("error out"=w318:errorcluster)  [unwired: 6 in, 1 out]
        n135 = call <userlib>:"CSM - Mark All Temp Variables as Permanent.vi"("error in (no error)"=w318) -> ("error out"=w317:errorcluster)  [unwired: 8 in]
        n136 = disable-structure shown="Enabled" {
          disable-tunnel: w324 -> [w333 _]
          disable-tunnel: w323 -> [w332 _]
          disable-tunnel: [w331 _] -> w322
          frame Disabled {
            n137 = call "Clean Layout.vi"("error in (no error)"=w333, "TabCtls"=w332) -> ("error out"=w331:errorcluster)  [unwired: 9 in]
          }
          frame Enabled {
          }
        }
        n138 = call <userlib>:"CSM - Sync Configuration Variables to File.vi"("Write UnSupported Datatype?(F)"=w319, "All Temp Variable to Default Ini(F)"=w319, "error in (no error)"=w317) -> ()  [unwired: 6 in, 1 out]
        n139 = Close Reference(reference=w328, error in (no error)=w322) -> (error out=w327:errorcluster)
        n140 = call <vilib>:"Add State(s) to Queue__JKI_lib_State_Machine.vi"("State(s) in (\"\")"=w330) -> ("States Out"=w329:string)  [unwired: 14 in]
      }
      frame "---------- Events ----------" {
        # "#CSM \"Category Seperator\"\nDo not put any code in this frame."
        n141 = call <vilib>:"Add State(s) to Queue__JKI_lib_State_Machine.vi"("State(s) in (\"\")"=w337) -> ("States Out"=w336:string)  [unwired: 14 in]
      }
      frame "Events: Register" {
        w341 = cluster{"TabCtl":refnum<vi>[]} {"TabCtl"=[]}  # TabCtlEvent
        # "#CSM \"Events: Register\"\nRegister user event. New Message Event is registered to break CSM waiting in event structure by default."
        # "#CSM Register New Message Event\nRegister message event to break Waiting in Event structure."
        n142 = Unbundle By Name(w339) -> ("1.Ref.TabCtls"=w338:refnum<vi>[])
        n143 = Bundle By Name(cluster=w341, "TabCtl"=w338) -> (w340:cluster{"TabCtl":refnum<vi>[]})
        n144 = call <userlib>:"CSM - Get New State Notifier Event.vi"("Name (\"\" to Use UUID)"=w345) -> ("error out"=w343:errorcluster, "New State Notifier Event"=w344:refnum<user-event>)  [unwired: 9 in]
        n145 = register-events(error in=w343, w344, w340, w340, w340) -> (reference out=w346:refnum<event-registration>, error out=w342:errorcluster)  [unwired: 1 in]
      }
      frame "Events: Unregister" {
        # "#CSM \"Events: Unregister\"\nUnregister user event."
        n146 = Unregister For Events(event registration refnum=w348) -> (error out=w349:errorcluster)  [unwired: 1 in]
      }
      frame "---------- UI ----------" {
        # "#CSM \"Category Seperator\"\nDo not put any code in this frame."
        n147 = call <vilib>:"Add State(s) to Queue__JKI_lib_State_Machine.vi"("State(s) in (\"\")"=w355) -> ("States Out"=w354:string)  [unwired: 14 in]
      }
      frame "UI: Initialize" {
        # "#CSM \"UI: Initialize\"\nInitialize the User Interface, here.\n(this is called automatically, by the Macro: Init)"
        n148 = call <vilib>:"Add State(s) to Queue__JKI_lib_State_Machine.vi"("State(s) in (\"\")"=w359) -> ("States Out"=w358:string)  [unwired: 14 in]
      }
      frame "UI: Save Layout" {
        n149 = Unbundle By Name(w367) -> ("1.Ref.TabCtls"=w364:refnum<vi>[], "1.Ref.Pane"=w363:refnum<vi>, "1.Val.LayoutMap"=w362:map{string, T4})
        n150 = Bundle By Name(cluster=T13 {"TabCtl"=[], "Pane"=refnum, "Variant"=variant, "map in"={}} ("input cluster"), "TabCtl"=w364, "Pane"=w363, "map in"=w362) -> (w365:T13)
        n151 = call "Save Layout.vi"("error in (no error)"=w370, "key"=w368, "input cluster"=w365) -> ("error out"=w369:errorcluster, "map out"=w360:map{string, T4})  [unwired: 7 in]
        n152 = Bundle By Name(cluster=w367, "1.Val.LayoutMap"=w360) -> (w361:T10)
      }
      frame "UI: Load Layout" {
        n153 = Unbundle By Name(w382) -> ("1.Ref.Pane"=w381:refnum<vi>, "1.Ref.TabCtls"=w380:refnum<vi>[], "1.Val.LayoutMap"=w379:map{string, T4}, "1.Val.ViewMap"=w373:map{string, T7})
        n154 = Bundle By Name(cluster=T14 {"Pane"=refnum, "TabCtls"=[], "map in"={}, "Views"={}} ("Cluster"), "Pane"=w381, "TabCtls"=w380, "map in"=w379, "Views"=w373) -> (w374:T14)
        n155 = call "Load Layout By Name.vi"("error in (no error)"=w377, "key"=w378, "Cluster"=w374) -> ("error out"=w376:errorcluster)  [unwired: 8 in]
      }
      frame "UI: Cursor Set" {
        # "Argument"
        # "#CSM \"UI: Cursor Set\"\nSet and Unset Cursor Busy.\n(Usage: \"UI: Cursor Set >> Busy|Idle\")"
        n156 = disable-structure shown="Default" {
          disable-tunnel: [w392 _] -> w387
          disable-tunnel: w386 -> [w391 _]
          frame condition #0 (active) {
            n157 = case shown="\"Idle\", Default" w391 {
              tunnel: [w393 w394] -> w392
              frame "Idle", Default {
                n158 = call <vilib>:"Unset Busy.vi"() -> ("error out"=w393:errorcluster)  [unwired: 11 in]
              }
              frame "Busy" {
                n159 = call <vilib>:"Set Busy.vi"() -> ("error out"=w394:errorcluster)  [unwired: 10 in, 1 out]
              }
            }
          }
          frame condition #1 {
          }
        }
        n160 = call <vilib>:"Add State(s) to Queue__JKI_lib_State_Machine.vi"("State(s) in (\"\")"=w390) -> ("States Out"=w389:string)  [unwired: 14 in]
      }
      frame "UI: Front Panel State" {
        # "Argument"
        # "#CSM \"UI: Front Panel State\"\nSet Front Panel Open or Closed\n(Usage: \"UI: Front Panel State >> Open|Close\")"
        n161 = Unbundle By Name(w398) -> ("Core.Current VI Reference"=w397:refnum<vi>)
        n162 = case shown="\"Close\", \"Closed\"" w396 {
          tunnel: [w408 w421 w432 w444 w456] -> w399
          tunnel: w397 -> [w407 w419 w431 w443 w455]
          frame "Open", "Standard", Default {
            w402 = T11."Standard" ("State")
            n163 = property class="VI"(reference=w407) -> (reference out=w405:refnum<vi>, error out=w406:errorcluster, "FP.State"=w404:T11)  [unwired: 1 in]
            n164 = Not Equal?(x=w404, y=w402) -> (x != y?=w403:bool)
            n165 = case shown="True" w403 {
              tunnel: [w412 w414] -> w408
              tunnel: w406 -> [w411 w414]
              tunnel: w405 -> [w410 _]
              tunnel: w402 -> [w409 _]
              frame True {
                n166 = invoke class="VI" method="FP.Open"(reference=w410, error in=w411, "Activate"=TRUE, "State"=w409) -> (error out=w412:errorcluster)  [unwired: 1 in, 4 out]
              }
              frame False {
              }
            }
          }
          frame "Close", "Closed" {
            n167 = property class="VI"(reference=w419) -> (reference out=w418:refnum<vi>, error out=w420:errorcluster, "FP.State"=w416:T11)  [unwired: 1 in]
            n168 = Not Equal?(x=w416, y=T11."Closed" ("Front Panel Window:State")) -> (x != y?=w415:bool)
            n169 = case shown="True" w415 {
              tunnel: [w422 w425] -> w421
              tunnel: w420 -> [w422 w424]
              tunnel: w418 -> [_ w423]
              frame False {
              }
              frame True {
                n170 = invoke class="VI" method="FP.Close"(reference=w423, error in=w424) -> (error out=w425:errorcluster)  [unwired: 1 in, 2 out]
              }
            }
          }
          frame "Hidden", "Hide" {
            w426 = T11."Hidden" ("State")
            n171 = property class="VI"(reference=w431) -> (reference out=w429:refnum<vi>, error out=w430:errorcluster, "FP.State"=w428:T11)  [unwired: 1 in]
            n172 = Not Equal?(x=w428, y=w426) -> (x != y?=w427:bool)
            n173 = case shown="True" w427 {
              tunnel: [w436 w437] -> w432
              tunnel: w430 -> [w435 w437]
              tunnel: w429 -> [w434 _]
              tunnel: w426 -> [w433 _]
              frame True {
                n174 = invoke class="VI" method="FP.Open"(reference=w434, error in=w435, "State"=w433) -> (error out=w436:errorcluster)  [unwired: 2 in, 4 out]
              }
              frame False {
              }
            }
          }
          frame "Minimize", "Minimized" {
            w438 = T11."Minimized" ("State")
            n175 = property class="VI"(reference=w443) -> (reference out=w441:refnum<vi>, error out=w442:errorcluster, "FP.State"=w440:T11)  [unwired: 1 in]
            n176 = Not Equal?(x=w440, y=w438) -> (x != y?=w439:bool)
            n177 = case shown="False" w439 {
              tunnel: [w448 w449] -> w444
              tunnel: w442 -> [w447 w449]
              tunnel: w441 -> [w446 _]
              tunnel: w438 -> [w445 _]
              frame True {
                n178 = invoke class="VI" method="FP.Open"(reference=w446, error in=w447, "State"=w445) -> (error out=w448:errorcluster)  [unwired: 2 in, 4 out]
              }
              frame False {
              }
            }
          }
          frame "Maximize", "Maximized" {
            w450 = T11."Maximized" ("State")
            n179 = property class="VI"(reference=w455) -> (reference out=w453:refnum<vi>, error out=w454:errorcluster, "FP.State"=w452:T11)  [unwired: 1 in]
            n180 = Not Equal?(x=w452, y=w450) -> (x != y?=w451:bool)
            n181 = case shown="True" w451 {
              tunnel: [w460 w461] -> w456
              tunnel: w454 -> [w459 w461]
              tunnel: w453 -> [w458 _]
              tunnel: w450 -> [w457 _]
              frame True {
                n182 = invoke class="VI" method="FP.Open"(reference=w458, error in=w459, "State"=w457) -> (error out=w460:errorcluster)  [unwired: 2 in, 4 out]
              }
              frame False {
              }
            }
          }
        }
        n183 = call <vilib>:"Add State(s) to Queue__JKI_lib_State_Machine.vi"("State(s) in (\"\")"=w401) -> ("States Out"=w400:string)  [unwired: 14 in]
      }
      frame "---------- Macro ----------" {
        # "#CSM \"Category Seperator\"\nDo not put any code in this frame."
        n184 = call <vilib>:"Add State(s) to Queue__JKI_lib_State_Machine.vi"("State(s) in (\"\")"=w465) -> ("States Out"=w464:string)  [unwired: 14 in]
      }
      frame "Macro: Initialize" {
        w467 = "Data: Initialize\nInitialize Core Data\nUI: Initialize\nUI: Front Panel State >> Maximize\nEvents: Register\n//UI: Front Panel State >> Open"  # Data: Initialize Initialize Core Data UI: Initialize UI: Front Panel State >> Maximize Events: Register //UI: Front Panel State >> Open
        # "#CSM \"Macro: Initialize\"\nInitialization Macro (This is called once, when the VI starts)"
        n185 = call <vilib>:"Add State(s) to Queue__JKI_lib_State_Machine.vi"("State(s) in Front (\"\")"=w467, "State(s) in (\"\")"=w470) -> ("States Out"=w469:string)  [unwired: 13 in]
      }
      frame "Macro: Exit" {
        # "#CSM \"Macro: Exit\"\nExit Macro (This is called once, when the VI exits)"
        n186 = Unbundle By Name(w479) -> ("Core.Close Panel on Exit?"=w478:bool)
        n187 = Select(t="UI: Front Panel State >> Close", s=w478, f="") -> (s? t:f=w475:string)
        n188 = call <vilib>:"Add State(s) to Queue__JKI_lib_State_Machine.vi"("State(s) in Front (\"\")"="//Exit Sub-Modules ", "State(s) in (\"\")"=w475, "State(s) at Back (\"\")"="Data: Cleanup\nEvents: Unregister\nExit") -> ("States Out"=w473:string)  [unwired: 12 in]
        n189 = call <vilib>:"Add State(s) to Queue__JKI_lib_State_Machine.vi"("State(s) in Front (\"\")"=w473, "State(s) in (\"\")"=w481) -> ("States Out"=w480:string)  [unwired: 13 in]
      }
      frame "---------- API ----------" {
        # "#CSM \"Category Seperator\"\nDo not put any code in this frame."
      }
      frame "API: Update View" {
        # "#CSM API Example\nCopy/Rename this case for your own API"
        n190 = call "Convert API String Arguments to Data.vim"("Reference Type"=T7 {"Name"="", "VIPath"=path "", "Height(Default)"=0, "Widht(Default)"=0, "VIRef"=refnum} ("value"), "API String"=w485) -> ("Data"=w486:T7)  [unwired: 6 in, 1 out]
        n191 = Unbundle By Name(w492) -> ("1.Val.ViewMap"=w491:map{string, T7})
        n192 = Unbundle By Name(w486) -> ("Name"=w487:string)
        n193 = Insert Into Map(map in=w491, key=w487, value=w486) -> (map out=w489:map{string, T7})  [unwired: 2 out]
        n194 = Bundle By Name(cluster=w492, "1.Val.ViewMap"=w489) -> (w490:T10)
      }
      frame "API: Update Subpanel" {
        w495 = refnum<vi> refnum  # SubPanel
        # "#CSM API Example\nCopy/Rename this case for your own API"
        n195 = Unbundle By Name(w504) -> ("Core.Current VI Reference"=w503:refnum<vi>)
        n196 = call "Convert API String Arguments to Data.vim"("Reference Type"=w495, "error in (no error)"=w499, "API String"=w496) -> ("error out"=w498:errorcluster, "Data"=w501:refnum<vi>)  [unwired: 5 in]
        n197 = property class="SubPnl"(reference=w501) -> ("OwningVI"=w500:refnum<vi>)  [unwired: 1 in, 2 out]
        n198 = invoke on="Invoke Node" class="VI" method="FP.Close"(reference=w503, error in=w498) -> (reference out=w505:refnum<vi>, error out=w506:errorcluster)  [unwired: 1 in, 1 out]
        n199 = invoke on="Invoke Node" class="SubPnl" method="Insert VI"(reference=w501, error in=w506, "VI Ref"=w505) -> (error out=w497:errorcluster)  [unwired: 1 in, 3 out]
        n200 = Bundle By Name(cluster=w504, "1.Ref.Owning VI"=w500) -> (w502:T10)
      }
      frame "API: Load Layout" {
        n201 = call <vilib>:"Build State String with Arguments__JKI_lib_State_Machine.vi"("Arguments (\"\")"=w512, "State"="UI: Load Layout") -> ("State with Arguments"=w509:string)  [unwired: 4 in]
        n202 = call <vilib>:"Add State(s) to Queue__JKI_lib_State_Machine.vi"("State(s) in Front (\"\")"=w509, "State(s) in (\"\")"=w511) -> ("States Out"=w510:string)  [unwired: 13 in]
      }
      frame "API: Save Layout" {
        n203 = call <vilib>:"Build State String with Arguments__JKI_lib_State_Machine.vi"("Arguments (\"\")"=w520, "State"="UI: Save Layout") -> ("State with Arguments"=w517:string)  [unwired: 4 in]
        n204 = call <vilib>:"Add State(s) to Queue__JKI_lib_State_Machine.vi"("State(s) in Front (\"\")"=w517, "State(s) in (\"\")"=w519) -> ("States Out"=w518:string)  [unwired: 13 in]
      }
      frame "---------- Action ----------" {
        # "#CSM \"Category Seperator\"\nDo not put any code in this frame."
        n205 = call <vilib>:"Add State(s) to Queue__JKI_lib_State_Machine.vi"("State(s) in (\"\")"=w528) -> ("States Out"=w527:string)  [unwired: 14 in]
      }
      frame "Action: action1" {
        # "#CSM \"Internal State\"\nThis category is used for holding internal states"
        n206 = call <vilib>:"Add State(s) to Queue__JKI_lib_State_Machine.vi"("State(s) in (\"\")"=w532) -> ("States Out"=w531:string)  [unwired: 14 in]
      }
      frame "Action: action2" {
        # "#CSM \"Internal State\"\nThis category is used for holding internal states"
        n207 = call <vilib>:"Add State(s) to Queue__JKI_lib_State_Machine.vi"("State(s) in (\"\")"=w536) -> ("States Out"=w535:string)  [unwired: 14 in]
      }
    }
  }
